vi "Read EtherCAT.vi"(8 "error in (no error)":errorcluster, 11 "RSI Module in":refnum<class "RSI Module.lvclass">) -> (0 "error out":errorcluster, 2 "EtherCAT?":bool, 3 "RSI Module out":refnum<class "RSI Module.lvclass">)   [LabVIEW 2020, in "Modules.lvlib" / "RSI Module.lvclass"]
uses:
  RSI Module.lvclass
  RSI Module.lvclass/RSI Module.ctl
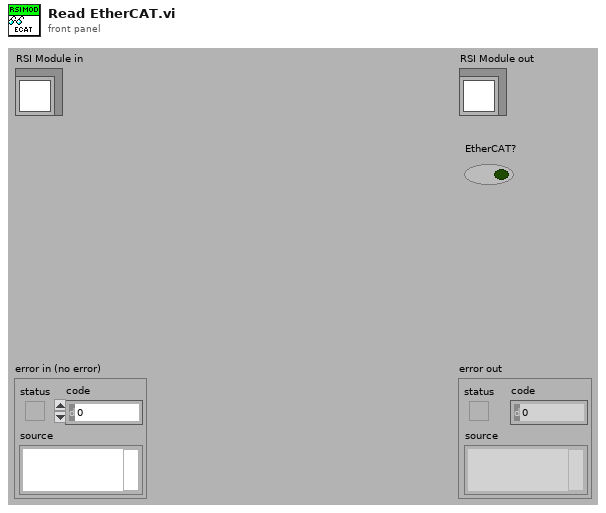
[diagram p1: front panel]
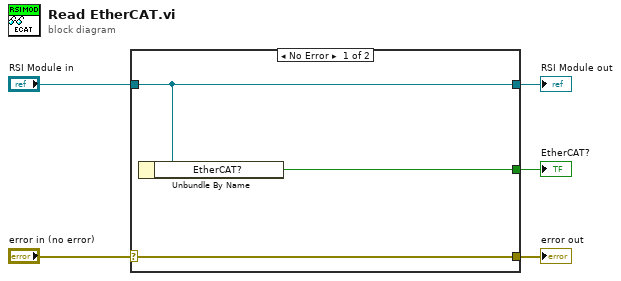
[diagram p0: block diagram]
diagram:
  n1 = case shown="No Error" "error in (no error)" {
    selector: "error in (no error)" -> [w8 w9]
    tunnel: [w8 w9] -> w4
    tunnel: [w7 w10] -> w2
    tunnel: "RSI Module in" -> [w7 w10]
    tunnel: [w6 _] -> w1
    frame No Error {
      n2 = Unbundle By Name(w7) -> ("EtherCAT?"=w6:bool)
    }
    frame Error {
    }
  }
  "error out" <- w4
  "RSI Module out" <- w2
  "EtherCAT?" <- w1
